vi "Queue Driver.vi"(0 "Queue Name":string, 5 "Enqueue Element":T1, 7 "Array of Elements":T1[](array[typedef]), 11 "Error In":errorcluster, 13 "Queue Operation":T2) -> (4 "Dequeue Element":T1, 15 "Error Out":errorcluster)   [LabVIEW 2019]
doc: "The VI performs the queue operations. The operations include create, enqueue, dequeue, flush and closes the queue."
uses:
  Controls/Queue Element.ctl
  Controls/Queue Operation.ctl
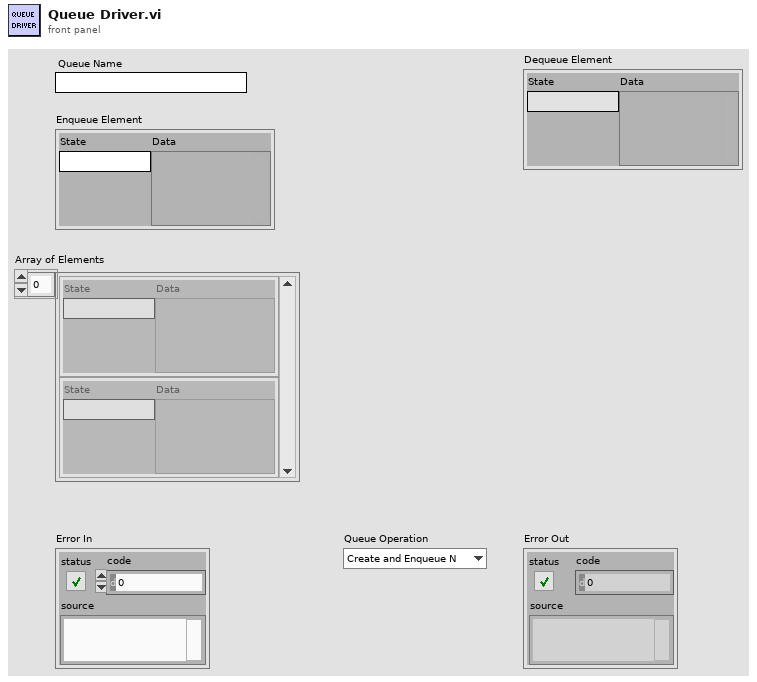
[diagram p1: front panel]
types:
  T1 = typedef "Queue Element.ctl" = cluster{"State":string, "Data":variant}
  T2 = typedef "Queue Operation.ctl" = enum16{"Create and Enqueue N", "Enqueue", "Enqueue N", "Dequeue", "Enstack N", "Flush", "Release"}
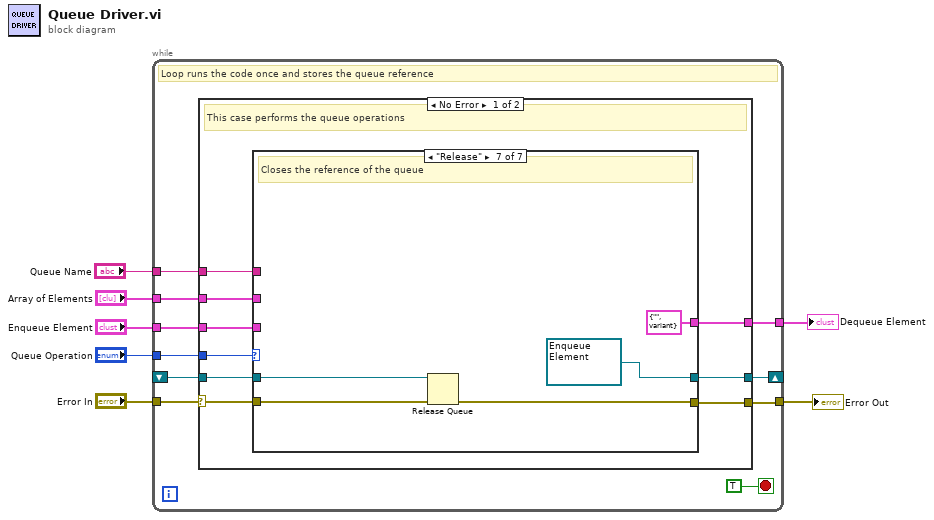
[diagram p0: block diagram]
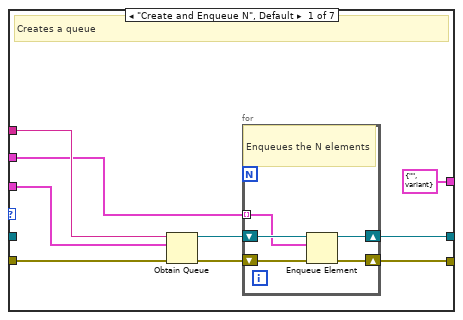
[diagram p2: hidden frame]
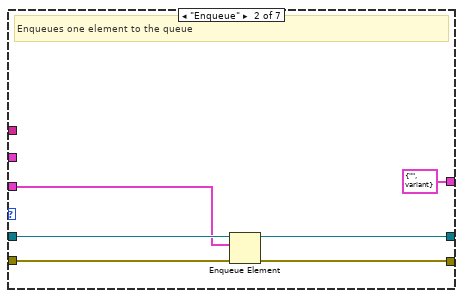
[diagram p3: hidden frame]
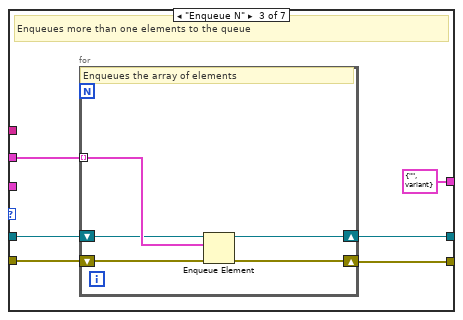
[diagram p4: hidden frame]
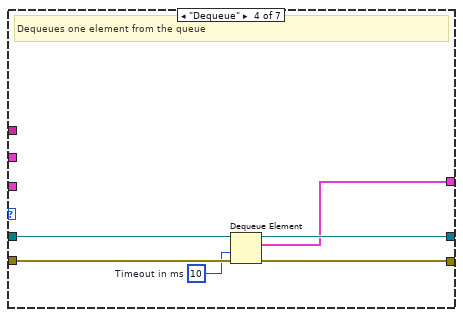
[diagram p5: hidden frame]
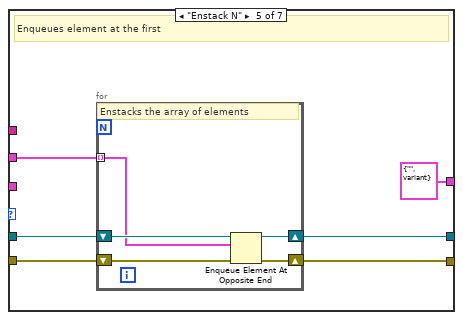
[diagram p6: hidden frame]
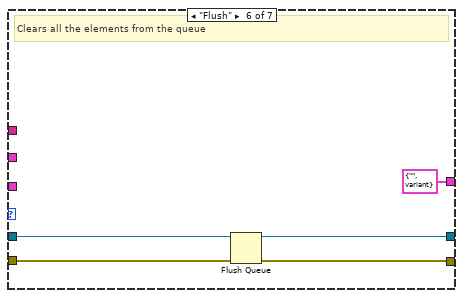
[diagram p7: hidden frame]
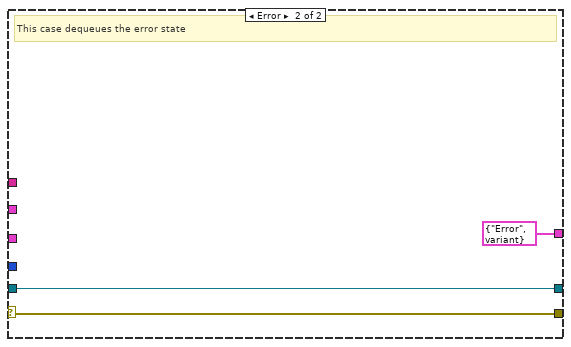
[diagram p8: hidden frame]
diagram:
  n1 = while {
    tunnel: "Queue Operation" -> [w16]
    tunnel: "Enqueue Element" -> [w15]
    tunnel: "Array of Elements" -> [w14]
    shift-right: [w13] -> _
    shift-left: _ -> [w12]
    tunnel: [w9] -> w2
    tunnel: "Queue Name" -> [w8]
    tunnel: "Error In" -> [w17]
    tunnel: [w11] -> w4
    stop <- TRUE stop-if-true
    # "Loop runs the code once and stores the queue reference"
    n2 = case shown="No Error" w17 {
      selector: w17 -> [w26 w86]
      tunnel: w16 -> [w25 _]
      tunnel: w15 -> [w24 _]
      tunnel: w14 -> [w23 _]
      tunnel: [w22 w87] -> w13
      tunnel: w12 -> [w21 w87]
      tunnel: [w20 w86] -> w11
      tunnel: [w19 T1 {"State"="Error", "Data"=variant} ("Enqueue Element")] -> w9
      tunnel: w8 -> [w18 _]
      frame No Error {
        # "This case performs the queue operations"
        n3 = case shown="\"Release\"" w25 {
          tunnel: [w30 w45 w51 w62 w68 w78 w83] -> w20
          tunnel: w26 -> [w35 w46 w52 w63 w69 w79 w84]
          tunnel: w24 -> [w33 w43 _ _ _ _ _]
          tunnel: w23 -> [w27 _ w50 _ w64 _ _]
          tunnel: [w28 w42 w48 w61 w66 w76 refnum<queue> refnum ("queue out")] -> w22
          tunnel: w21 -> [_ w44 w49 w60 w67 w77 w82]
          tunnel: [T1 {"State"="", "Data"=variant} ("Enqueue Element") T1 {"State"="", "Data"=variant} ("Enqueue Element") T1 {"State"="", "Data"=variant} ("Enqueue Element") w58 T1 {"State"="", "Data"=variant} ("Enqueue Element") T1 {"State"="", "Data"=variant} ("Enqueue Element") T1 {"State"="", "Data"=variant} ("Enqueue Element")] -> w19
          tunnel: w18 -> [w31 _ _ _ _ _ _]
          frame "Create and Enqueue N", Default {
            # "Creates a queue"
            n4 = Obtain Queue(name (unnamed)=w31, element data type=w33, error in (no error)=w35) -> (queue out=w29:refnum<queue>, error out=w34:errorcluster)  [unwired: 2 in, 1 out]
            n5 = for {
              shift-right: [w39] -> w30
              shift-left: w34 -> [w40]
              shift-right: [w37] -> w28
              shift-left: w29 -> [w38]
              tunnel: w27 -> [w36] mode=indexing
              # "Enqueues the N elements"
              n6 = Enqueue Element(queue=w38, element=w36, error in (no error)=w40) -> (queue out=w37:refnum<queue>, error out=w39:errorcluster)  [unwired: 1 in, 1 out]
            }
          }
          frame "Enqueue" {
            # "Enqueues one element to the queue"
            n7 = Enqueue Element(queue=w44, element=w43, error in (no error)=w46) -> (queue out=w42:refnum<queue>, error out=w45:errorcluster)  [unwired: 1 in, 1 out]
          }
          frame "Enqueue N" {
            # "Enqueues more than one elements to the queue"
            n8 = for {
              shift-right: [w56] -> w51
              shift-left: w52 -> [w57]
              tunnel: w50 -> [w55] mode=indexing
              shift-right: [w53] -> w48
              shift-left: w49 -> [w54]
              # "Enqueues the array of elements"
              n9 = Enqueue Element(queue=w54, element=w55, error in (no error)=w57) -> (queue out=w53:refnum<queue>, error out=w56:errorcluster)  [unwired: 1 in, 1 out]
            }
          }
          frame "Dequeue" {
            w59 = 10  # Timeout in ms
            # "Dequeues one element from the queue"
            n10 = Dequeue Element(queue=w60, timeout in ms (-1)=w59, error in (no error)=w63) -> (queue out=w61:refnum<queue>, element=w58:T1, error out=w62:errorcluster)  [unwired: 1 out]
          }
          frame "Enstack N" {
            # "Enqueues element at the first"
            n11 = for {
              shift-right: [w73] -> w68
              shift-left: w69 -> [w74]
              shift-right: [w71] -> w66
              shift-left: w67 -> [w72]
              tunnel: w64 -> [w70] mode=indexing
              # "Enstacks the array of elements"
              n12 = Enqueue Element At Opposite End(queue=w72, element=w70, error in (no error)=w74) -> (queue out=w71:refnum<queue>, error out=w73:errorcluster)  [unwired: 1 in, 1 out]
            }
          }
          frame "Flush" {
            # "Clears all the elements from the queue"
            n13 = Flush Queue(queue=w77, error in (no error)=w79) -> (queue out=w76:refnum<queue>, error out=w78:errorcluster)  [unwired: 1 out]
          }
          frame "Release" {
            # "Closes the reference of the queue"
            n14 = Release Queue(queue=w82, error in (no error)=w84) -> (error out=w83:errorcluster)  [unwired: 1 in, 2 out]
          }
        }
      }
      frame Error {
        # "This case dequeues the error state"
      }
    }
  }
  "Error Out" <- w4
  "Dequeue Element" <- w2
